vi "Rohde_Measure_PS.vi"(8 "error in (no error)":errorcluster, 10 "Channel":i32(ring)=1 caption="Channel (Channel 1)" items=["Channel 1"=1, "Channel 2"=2, "Channel 3"=3, "Channel 4"=4]) -> (0 "error out":errorcluster, 2 "Current (A)":dbl caption="Current Value" format="%.3f", 3 "Voltage (V)":dbl caption="Voltage Value" format="%.3f")   [LabVIEW 2018]
panel:
  out "PsV&I":string
  out "PsAddressOut":refnum<visa-resource-name> caption="VISA resource name out"
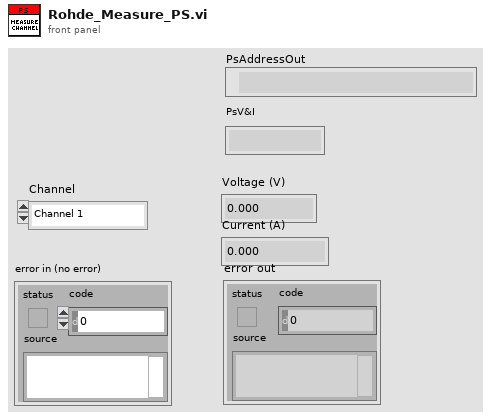
[diagram p1: front panel]
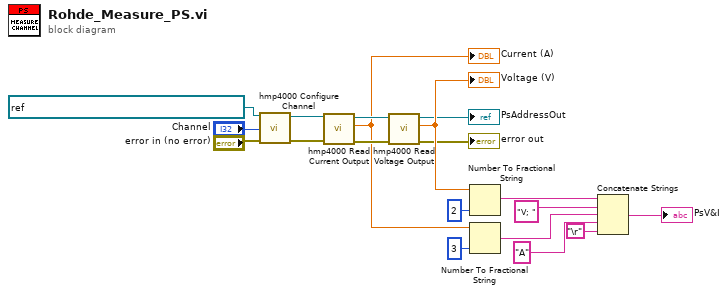
[diagram p0: block diagram]
diagram:
  n1 = call "hmp4000 Configure Channel.vi"("error in (no error)"="error in (no error)", "Channel (Channel 1)"="Channel", "VISA resource name"=refnum<visa-resource-name> "TCPIP::10.42.0.201::5025::SOCKET") -> ("error out"=w10:errorcluster, "VISA resource name out"=w11:refnum<visa-resource-name>)  [unwired: 7 in]
  n2 = call "hmp4000 Read Current Output.vi"("error in (no error)"=w10, "VISA resource name"=w11) -> ("error out"=w13:errorcluster, "Current Value"=w7:dbl, "VISA resource name out"=w12:refnum<visa-resource-name>)  [unwired: 7 in]
  "Current (A)" <- w7
  n3 = call "hmp4000 Read Voltage Output.vi"("error in (no error)"=w13, "VISA resource name"=w12) -> ("error out"=→"error out":errorcluster, "Voltage Value"=w14:dbl, "VISA resource name out"=→"PsAddressOut":refnum<visa-resource-name>)  [unwired: 7 in]
  "Voltage (V)" <- w14
  n4 = Number To Fractional String(number=w14, precision (6)=i16 2) -> (F-format string=w15:string)  [unwired: 2 in]
  n5 = Number To Fractional String(number=w7, precision (6)=i16 3) -> (F-format string=w8:string)  [unwired: 2 in]
  n6 = Concatenate Strings(w15, "V; ", w8, "A", "\r") -> (→"PsV&I":string)
